vi "ini_object_load.vi"(7 "generate error if unsuppoted data type (true)":bool=TRUE, 8 "error in":errorcluster, 10 "auto ini row":T1, 11 "refnum in":T2) -> (0 "error out":errorcluster, 3 "refnum out":T2)   [LabVIEW 2013]
uses:
  <vilib>/Utility/config.llb/Config Data RefNum.ctl
  ini_parse_row.ctl
  <vilib>/Utility/config.llb/Read Key (String).vi
  <vilib>/regexp/Match Regular Expression.xnode
  <vilib>/Utility/config.llb/NI_LVConfig.lvlib
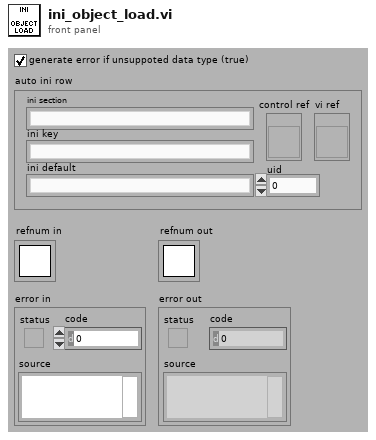
[diagram p1: front panel]
types:
  T1 = typedef "ini_parse_row.ctl" = cluster{"ini section":string, "ini key":string, "ini default":string, "control ref":refnum<vi>, "uid":i32, "vi ref":refnum<vi>}
  T2 = typedef "NI_LVConfig.lvlib/Config Data RefNum.ctl" = refnum<k1>
  T3 = cluster{"Value":string[][], "Row Headers[]":string[], "Column Headers[]":string[]}
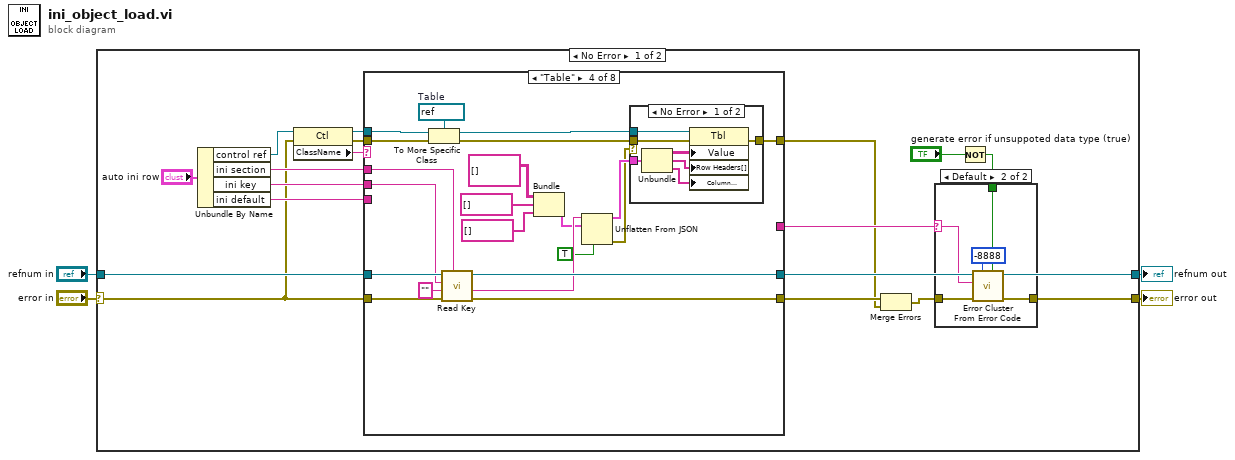
[diagram p0: block diagram]
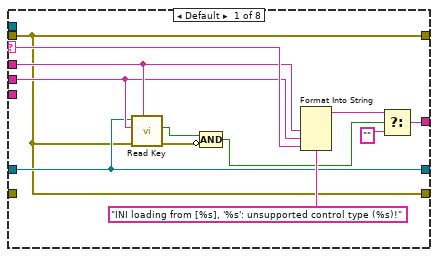
[diagram p3: hidden frame]
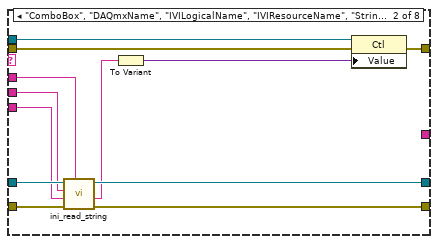
[diagram p4: hidden frame]
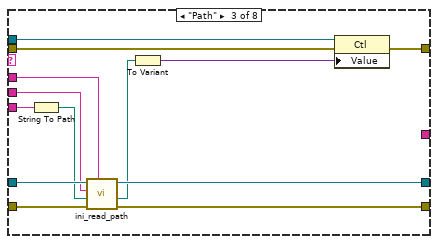
[diagram p5: hidden frame]
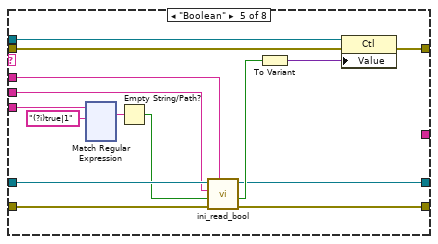
[diagram p7: hidden frame]
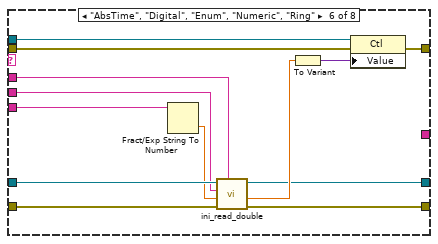
[diagram p8: hidden frame]
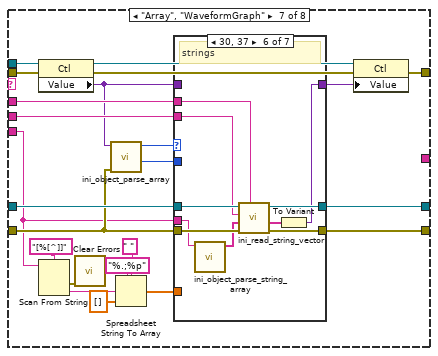
[diagram p9: hidden frame]
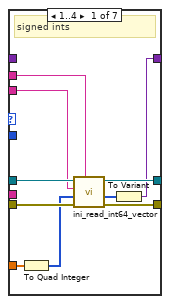
[diagram p10: hidden frame]
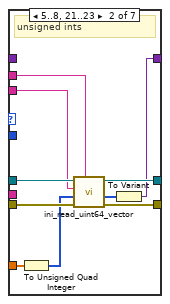
[diagram p11: hidden frame]
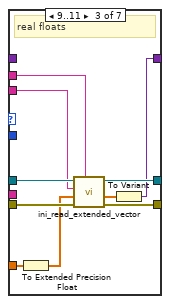
[diagram p12: hidden frame]
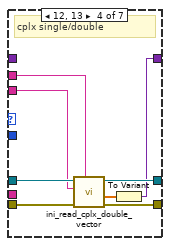
[diagram p13: hidden frame]
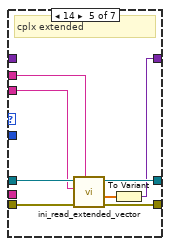
[diagram p14: hidden frame]
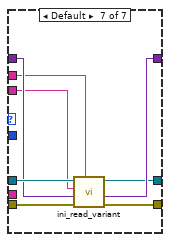
[diagram p15: hidden frame]
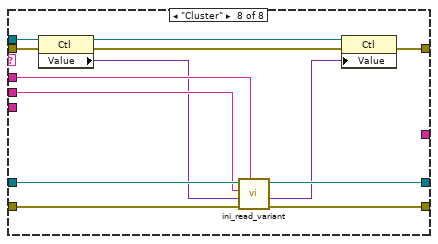
[diagram p16: hidden frame]
diagram:
  n1 = case shown="No Error" "error in" {
    selector: "error in" -> [w6 w338]
    tunnel: "refnum in" -> [w22 w337]
    tunnel: [w21 w337] -> w3
    tunnel: [w12 w338] -> w2
    frame No Error {
      n2 = Unbundle By Name("auto ini row") -> ("control ref"=w17:refnum<vi>, "ini section"=w19:string, "ini key"=w18:string, "ini default"=w15:string)
      n3 = property class="Ctl"(reference=w17, error in=w6) -> (reference out=w13:refnum<vi>, error out=w14:errorcluster, "ClassName"=w16:string)
      n4 = case shown="\"Table\"" w16 {
        selector: w16 -> [w39 _ _ _ _ _ _ _]
        tunnel: [w29 w49 w62 w83 w100 w229 w256 w333] -> w8
        tunnel: w22 -> [w30 w51 w64 w85 w107 w235 w259 w336]
        tunnel: [w30 w50 w63 w84 w99 w228 w255 w332] -> w21
        tunnel: w19 -> [w32 w48 w61 w82 w106 w234 w258 w335]
        tunnel: w18 -> [w31 w47 w60 w81 w105 w233 w257 w334]
        tunnel: w15 -> [_ w46 w59 _ w104 w232 w241 _]
        tunnel: w14 -> [w29 w44 w55 w79 w98 w227 w247 w331]
        tunnel: w13 -> [_ w43 w53 w78 w97 w225 w246 w330]
        tunnel: [w36 _ _ _ _ _ _ _] -> w11
        tunnel: w6 -> [_ w52 w65 w86 w108 w236 w245 w329]
        tunnel: [w29 w42 w56 w80 w95 w226 w240 w327] -> w5
        frame Default {
          n5 = call-poly <vilib>:"Read Key.vi"("section"=w32, "error in (no error)"=w29, "key"=w31, "refnum"=w30) -> ("error out"=w37:errorcluster, "found?"=w38:bool)  [unwired: 4 in, 2 out]
          n6 = Compound Arithmetic op=AND(w38, invert w37) -> (w35:bool)
          n7 = Format Into String(format string="INI loading from [%s], '%s': unsupported control type (%s)!", w32, w31, w39) -> (resulting string=w34:string)  [unwired: 2 in, 1 out]
          n8 = Select(t=w34, s=w35, f="") -> (s? t:f=w36:string)
        }
        frame "ComboBox", "DAQmxName", "IVILogicalName", "IVIResourceName", "String", "VISAResourceName" {
          n9 = call "ini_read_string.vi"("section"=w48, "error in"=w52, "default value"=w46, "key"=w47, "refnum in"=w51) -> ("error out"=w49:errorcluster, "value"=w45:string, "refnum out"=w50:T2)  [unwired: 3 in, 1 out]
          n10 = To Variant(anything=w45) -> (Variant=w41:variant)
          n11 = property class="Ctl"(reference=w43, error in=w44, "Value"=w41) -> (error out=w42:errorcluster)  [unwired: 1 out]
        }
        frame "Path" {
          n12 = String To Path(string=w59) -> (path=w57:path)
          n13 = call "ini_read_path.vi"("section"=w61, "error in"=w65, "default value"=w57, "key"=w60, "refnum in"=w64) -> ("error out"=w62:errorcluster, "value"=w58:path, "refnum out"=w63:T2)  [unwired: 3 in, 1 out]
          n14 = To Variant(anything=w58) -> (Variant=w54:variant)
          n15 = property class="Ctl"(reference=w53, error in=w55, "Value"=w54) -> (error out=w56:errorcluster)  [unwired: 1 out]
        }
        frame "Table" {
          w75 = refnum<vi> refnum  # Table
          n16 = To More Specific Class(target class=w75, reference=w78, error in=w79) -> (specific class reference=w77:refnum<vi>, error out=w76:errorcluster)
          n17 = call-poly <vilib>:"Read Key.vi"("section"=w82, "error in (no error)"=w86, "default value"="", "key"=w81, "refnum"=w85) -> ("error out"=w83:errorcluster, "value"=w72:string, "refnum out"=w84:T2)  [unwired: 3 in, 1 out]
          n18 = Bundle("Value"=string[][] [], "Row Headers[]"=string[] [], "Column Headers[]"=string[] []) -> (w66:T3)  [unwired: 1 in]
          n19 = Unflatten From JSON(JSON string=w72, type and defaults=w66, default null elements? (F)=TRUE) -> (value=w74:T3, error out=w71:errorcluster)  [unwired: 4 in]
          n20 = case shown="No Error" w71 {
            tunnel: [w93 w94] -> w80
            tunnel: w77 -> [w92 _]
            tunnel: w76 -> [w91 w94]
            tunnel: w74 -> [w90 _]
            frame No Error {
              n21 = Unbundle(w90) -> ("Value"=w89:string[][], "Row Headers[]"=w88:string[], "Column Headers[]"=w87:string[])
              n22 = property class="Tbl"(reference=w92, error in=w91, "Value"=w89, "Row Headers[]"=w88, "Column Headers[]"=w87) -> (error out=w93:errorcluster)  [unwired: 1 out]
            }
            frame Error {
            }
          }
        }
        frame "Boolean" {
          n23 = xnode "Match Regular Expression"("input string"=w104, "regular expression"="(?i)true|1") -> ("whole match"=w102:string)  [unwired: 4 in, 4 out]
          n24 = Empty String/Path?(string/path=w102) -> (empty?=w101:bool)
          n25 = call "ini_read_bool.vi"("section"=w106, "error in"=w108, "default value"=w101, "key"=w105, "refnum in"=w107) -> ("error out"=w100:errorcluster, "value"=w109:bool, "refnum out"=w99:T2)  [unwired: 3 in, 1 out]
          n26 = To Variant(anything=w109) -> (Variant=w96:variant)
          n27 = property class="Ctl"(reference=w97, error in=w98, "Value"=w96) -> (error out=w95:errorcluster)  [unwired: 1 out]
        }
        frame "AbsTime", "Digital", "Enum", "Numeric", "Ring" {
          n28 = Fract/Exp String To Number(string=w232) -> (number=w231:dbl)  [unwired: 3 in, 1 out]
          n29 = call "ini_read_double.vi"("section"=w234, "error in"=w236, "default value"=w231, "key"=w233, "refnum in"=w235) -> ("error out"=w229:errorcluster, "value"=w230:dbl, "refnum out"=w228:T2)  [unwired: 3 in, 1 out]
          n30 = To Variant(anything=w230) -> (Variant=w224:variant)
          n31 = property class="Ctl"(reference=w225, error in=w227, "Value"=w224) -> (error out=w226:errorcluster)  [unwired: 1 out]
        }
        frame "Array", "WaveformGraph" {
          n32 = property class="Ctl"(reference=w246, error in=w247) -> (reference out=w239:refnum<vi>, error out=w237:errorcluster, "Value"=w243:variant)
          n33 = Scan From String(format string="[%[^]]", input string=w241) -> (error out=w249:errorcluster, output 1=w253:string)  [unwired: 3 in, 2 out]
          n34 = call <vilib>:"Clear Errors.vi"("error in (no error)"=w249) -> ()  [unwired: 6 in, 1 out]
          n35 = call "ini_object_parse_array.vi"("error in"=w245, "variant in"=w243) -> ("dims"=w242:i16, "type id"=w244:i16)  [unwired: 6 in, 2 out]
          n36 = Spreadsheet String To Array(delimiter (Tab)=" ", format string="%.;%p", spreadsheet string=w253, array type (2D Dbl)=ext[] []) -> (array=w248:ext[])
          n37 = case shown="30, 37" w244 {
            tunnel: w259 -> [w269 w279 w289 w297 w305 w315 w319]
            tunnel: w258 -> [w268 w278 w288 w296 w304 w314 w317]
            tunnel: w257 -> [w267 w277 w287 w295 w303 w313 w316]
            tunnel: [w262 w272 w282 w291 w299 w309 w322] -> w238
            tunnel: [w266 w276 w286 w294 w302 w312 w321] -> w256
            tunnel: [w265 w275 w285 w293 w301 w311 w320] -> w255
            tunnel: w248 -> [w264 w274 w284 _ _ _ _]
            tunnel: w245 -> [w263 w273 w283 w292 w300 w310 w323]
            tunnel: w243 -> [_ _ _ _ _ _ w318]
            tunnel: w242 -> [_ _ _ _ _ _ _]
            tunnel: w241 -> [_ _ _ _ _ w306 _]
            frame 1..4 {
              # "signed ints"
              n38 = To Quad Integer(1:w264) -> (0:w260:i64[])
              n39 = call "ini_read_int64_vector.vi"("section"=w268, "error in"=w263, "default"=w260, "key"=w267, "refnum in"=w269) -> ("error out"=w266:errorcluster, "values"=w261:i64[], "refnum out"=w265:T2)  [unwired: 3 in, 1 out]
              n40 = To Variant(anything=w261) -> (Variant=w262:variant)
            }
            frame 5..8, 21..23 {
              # "unsigned ints"
              n41 = To Unsigned Quad Integer(1:w274) -> (0:w270:u64[])
              n42 = call "ini_read_uint64_vector.vi"("section"=w278, "error in"=w273, "default"=w270, "key"=w277, "refnum in"=w279) -> ("error out"=w276:errorcluster, "values"=w271:u64[], "refnum out"=w275:T2)  [unwired: 3 in, 1 out]
              n43 = To Variant(anything=w271) -> (Variant=w272:variant)
            }
            frame 9..11 {
              # "real floats"
              n44 = To Extended Precision Float(1:w284) -> (0:w280:ext[])
              n45 = call "ini_read_extended_vector.vi"("section"=w288, "error in"=w283, "default"=w280, "key"=w287, "refnum in"=w289) -> ("error out"=w286:errorcluster, "values"=w281:ext[], "refnum out"=w285:T2)  [unwired: 3 in, 1 out]
              n46 = To Variant(anything=w281) -> (Variant=w282:variant)
            }
            frame 12, 13 {
              # "cplx single/double"
              n47 = call "ini_read_cplx_double_vector.vi"("section"=w296, "error in"=w292, "key"=w295, "refnum in"=w297) -> ("error out"=w294:errorcluster, "values"=w290:cdb[], "refnum out"=w293:T2)  [unwired: 4 in, 1 out]
              n48 = To Variant(anything=w290) -> (Variant=w291:variant)
            }
            frame 14 {
              # "cplx extended"
              n49 = call "ini_read_extended_vector.vi"("section"=w304, "error in"=w300, "key"=w303, "refnum in"=w305) -> ("error out"=w302:errorcluster, "values"=w298:ext[], "refnum out"=w301:T2)  [unwired: 4 in, 1 out]
              n50 = To Variant(anything=w298) -> (Variant=w299:variant)
            }
            frame 48, 55 {
              # "strings"
              n51 = call "ini_object_parse_string_array.vi"("string in"=w306) -> ("string array out"=w307:string[])  [unwired: 9 in, 1 out]
              n52 = call "ini_read_string_vector.vi"("section"=w314, "error in"=w310, "default"=w307, "key"=w313, "refnum in"=w315) -> ("error out"=w312:errorcluster, "values"=w308:string[], "refnum out"=w311:T2)  [unwired: 3 in, 1 out]
              n53 = To Variant(anything=w308) -> (Variant=w309:variant)
            }
            frame Default {
              n54 = call "ini_read_variant.vi"("section"=w317, "error in"=w323, "default"=w318, "key"=w316, "refnum in"=w319) -> ("error out"=w321:errorcluster, "variant out"=w322:variant, "refnum out"=w320:T2)  [unwired: 3 in, 1 out]
            }
          }
          n55 = property class="Ctl"(reference=w239, error in=w237, "Value"=w238) -> (error out=w240:errorcluster)  [unwired: 1 out]
        }
        frame "Cluster" {
          n56 = property class="Ctl"(reference=w330, error in=w331) -> (reference out=w325:refnum<vi>, error out=w326:errorcluster, "Value"=w328:variant)
          n57 = call "ini_read_variant.vi"("section"=w335, "error in"=w329, "default"=w328, "key"=w334, "refnum in"=w336) -> ("error out"=w333:errorcluster, "variant out"=w324:variant, "refnum out"=w332:T2)  [unwired: 3 in, 1 out]
          n58 = property class="Ctl"(reference=w325, error in=w326, "Value"=w324) -> (error out=w327:errorcluster)  [unwired: 1 out]
        }
      }
      n59 = Merge Errors(w8, w5) -> (w7:errorcluster)
      n60 = Not(x="generate error if unsuppoted data type (true)") -> (.not. x?=w9:bool)
      n61 = case shown="Default" w11 {
        selector: w11 -> [_ w25]
        tunnel: w7 -> [w23 w28]
        tunnel: [w23 w27] -> w12
        tunnel: w9 -> [_ w24]
        frame "" {
        }
        frame Default {
          n62 = call <vilib>:"Error Cluster From Error Code.vi"("is warning? (False)"=w24, "error in (no error)"=w28, "error message (\"\")"=w25, "error code (0)"=-8888) -> ("error out"=w27:errorcluster)  [unwired: 5 in]
        }
      }
    }
    frame Error {
    }
  }
  "error out" <- w2
  "refnum out" <- w3
